vi "Create from VI.vi"(7 "Test Name":string, 8 "error in (no error)":errorcluster, 10 "Test Method VI Path":path, 11 "LUnit Test Case In":refnum<class "LUnit Test Case.lvclass">) -> (0 "error out":errorcluster, 3 "LUnit Test Case Out":refnum<class "LUnit Test Case.lvclass">)   [LabVIEW 2020, in "LUnit Test Case.lvclass"]
doc: "Create a test case object from a VI Path. Leave the test name unwired to use default."
uses:
  LUnit Test Case.lvclass
  LUnit Test Case.lvclass/LUnit Test Case.ctl
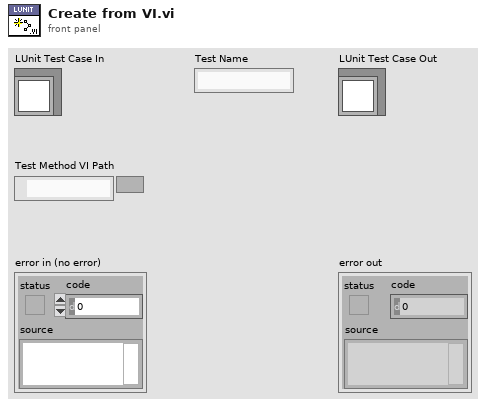
[diagram p1: front panel]
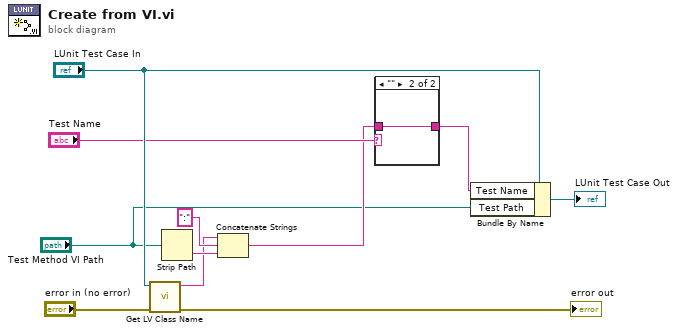
[diagram p0: block diagram]
diagram:
  n1 = call <vilib>:"Get LV Class Name.vi"("error in (no error)"="error in (no error)", "object"="LUnit Test Case In") -> ("error out"=→"error out":errorcluster, "class name"=w3:string)  [unwired: 8 in]
  n2 = Strip Path(path="Test Method VI Path") -> (name=w4:string)  [unwired: 1 out]
  n3 = Concatenate Strings(w3, ":" ("string"), w4) -> (w2:string)
  n4 = case shown="\"\"" "Test Name" {
    selector: "Test Name" -> [w12 _]
    tunnel: w2 -> [_ w13]
    tunnel: [w12 w13] -> w9
    frame Default {
    }
    frame "" {
    }
  }
  n5 = Bundle By Name(cluster="LUnit Test Case In", "Test Name"=w9, "Test Path"="Test Method VI Path") -> (→"LUnit Test Case Out":refnum<class "LUnit Test Case.lvclass">)
